vi "Auton Config File Read.vi"() -> (0 "GainSlow":dbl, 1 "Distance":dbl, 2 "Speed":dbl, 3 "GainFast":dbl)   [LabVIEW 2013]
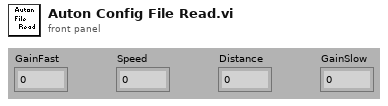
[diagram p1: front panel]
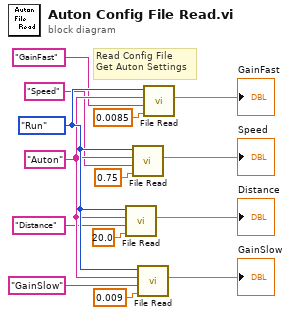
[diagram p0: block diagram]
diagram:
  w10 = "Auton" ("section")
  w11 = enum16{"Init", "Run", "End"}."Run" ("Mode")
  # "Read Config File\nGet Auton Settings"
  n1 = call "File Read.vi"("Default Value"=20.0, "key"="Distance", "section"=w10, "Mode"=w11) -> ("Output Value"=→"Distance":dbl)  [unwired: 7 out]
  n2 = call "File Read.vi"("Default Value"=0.75, "key"="Speed", "section"=w10, "Mode"=w11) -> ("Output Value"=→"Speed":dbl)  [unwired: 7 out]
  n3 = call "File Read.vi"("Default Value"=0.009, "key"="GainSlow", "section"=w10, "Mode"=w11) -> ("Output Value"=→"GainSlow":dbl)  [unwired: 7 out]
  n4 = call "File Read.vi"("Default Value"=0.0085, "key"="GainFast", "section"=w10, "Mode"=w11) -> ("Output Value"=→"GainFast":dbl)  [unwired: 7 out]
